vi "unit_converter.vi"   [LabVIEW 2017, in "sensor_translation.lvlib"]
uses:
  sensor_translation.lvlib
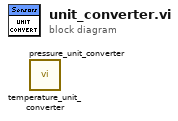
[diagram p0: block diagram]
diagram:
  n1 = call "temperature_unit_converter.vi"() -> ()  [unwired: 3 in, 1 out]
  n2 = call "pressure_unit_converter.vi"() -> ()  [unwired: 3 in, 1 out]
